vi "GetFileDatafromIndex.vi"(8 "Error In":errorcluster, 11 "DuplicateFilteredIndex":u32) -> (0 "Error Out":errorcluster, 1 "FreezeAbsTime":timestamp, 2 "FreezeFileName":string, 3 "FreezeTemperature":dbl format="%#_13g", 5 "Peak index":u32)   [LabVIEW 2015]
uses:
  DB/ConfDB.ctl
  TypeDef/Magnification.ctl
  DB/ConfEnum.ctl
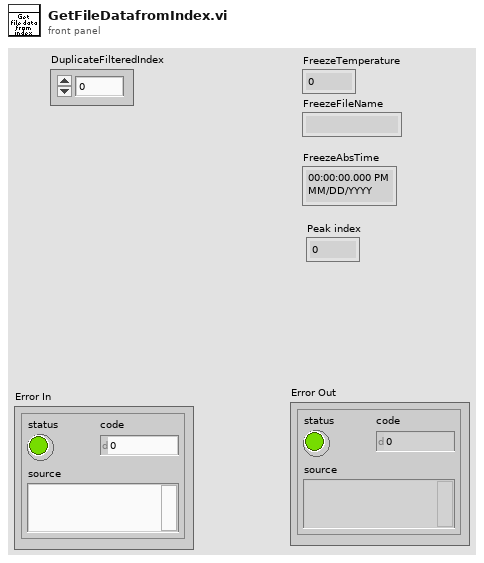
[diagram p1: front panel]
types:
  T1 = typedef "ConfEnum.ctl" = enum16{"Insert Threshold Freeze Score", "Insert TolXStd", "ReplacePath", "Init", "GetConfDB", "GetTemperatureAtIndex", "WriteConfDB", "InsertMagnification", "Configure DB"}
  T2 = typedef "ConfDB.ctl" = cluster{"NumberOfImages":i32, "Threshold Freeze score":i32, "Path":path, "NameOfPartialFile":string, "StartIndex":i32, "NumberOfStdTol":i32, "Detection Droplet Frame Index":i32, "Number of images for baseline":i32, "Temperature File Name":string, "Score":dbl, "Index number of Files":i32[], "End Index":i32, "Temperature Array":dbl[], "TStartIndex":i32, "Magnification (Microns/Pixel)":T3, "Circle Descriptor":cluster{"Min Radius":dbl, "Max Radius":dbl}}
  T3 = typedef "Magnification.ctl" = dbl
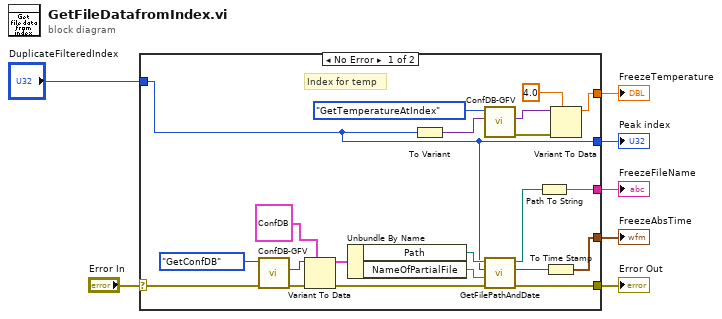
[diagram p0: block diagram]
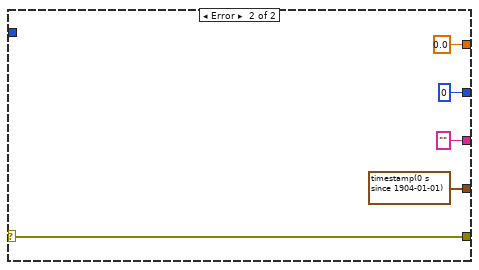
[diagram p2: hidden frame]
diagram:
  n1 = case shown="No Error" "Error In" {
    selector: "Error In" -> [w22 w33]
    tunnel: "DuplicateFilteredIndex" -> [w13 _]
    tunnel: [w18 w33] -> w5
    tunnel: [w19 timestamp(0 s since 1904-01-01)] -> w4
    tunnel: [w15 "" ("name")] -> w3
    tunnel: [w13 0] -> w2
    tunnel: [w8 0.0] -> w1
    frame No Error {
      # "Index for temp"
      n2 = call "ConfDB-GFV.vi"("error in (no error)"=w22, "Command In"=ConfEnum."GetConfDB") -> ("error out"=w25:errorcluster, "Data out"=w26:variant)  [unwired: 8 in]
      n3 = Variant To Data(error in=w25, type=T2 {"NumberOfImages"=0, "Threshold Freeze score"=0, "Path"=path "", "NameOfPartialFile"="", "StartIndex"=0, "NumberOfStdTol"=0, "Detection Droplet Frame Index"=0, "Number of images for baseline"=0, "Temperature File Name"="", "Score"=0.0, "Index number of Files"=[], "End Index"=0, "Temperature Array"=[], "TStartIndex"=0, "Magnification (Microns/Pixel)"=0.0, "Circle Descriptor"={"Min Radius"=0.0, "Max Radius"=0.0}} ("ConfDB"), Variant=w26) -> (data=w27:T2, error out=w21:errorcluster)
      n4 = Unbundle By Name(w27) -> ("Path"=w17:path, "NameOfPartialFile"=w28:string)
      n5 = To Variant(anything=w13) -> (Variant=w12:variant)
      n6 = call "ConfDB-GFV.vi"("Data in"=w12, "Command In"=ConfEnum."GetTemperatureAtIndex") -> ("error out"=w11:errorcluster, "Data out"=w10:variant)  [unwired: 8 in]
      n7 = call "GetFilePathAndDate.vi"("error in (no error)"=w21, "String"=w28, "Index"=w13, "Path"=w17) -> ("error out"=w18:errorcluster, "creation date"=w20:u32, "file out"=w16:path)  [unwired: 5 in]
      n8 = Path To String(path=w16) -> (string=w15:string)
      n9 = To Time Stamp(1:w20) -> (0:w19:timestamp)
      n10 = Variant To Data(error in=w11, type=4.0 ("disabled index (col)"), Variant=w10) -> (data=w8:dbl)  [unwired: 1 out]
    }
    frame Error {
    }
  }
  "Error Out" <- w5
  "FreezeTemperature" <- w1
  "FreezeFileName" <- w3
  "FreezeAbsTime" <- w4
  "Peak index" <- w2
